vi "makeLines.vi"(7 "d (mm)":dbl, 8 "error in (no error)":errorcluster, 9 "L (mm)":dbl, 10 "N Cycles":i32, 11 "VISA Refnum in":refnum<visa-resource-name>) -> (0 "error out":errorcluster, 3 "VISA Refnum out":refnum<visa-resource-name>)   [LabVIEW 2014]
doc: "Newport Motion Controler\nThis sub VI make lines structure\n\nAndré Romero - 2022\nandretec@ifsc.usp.br"
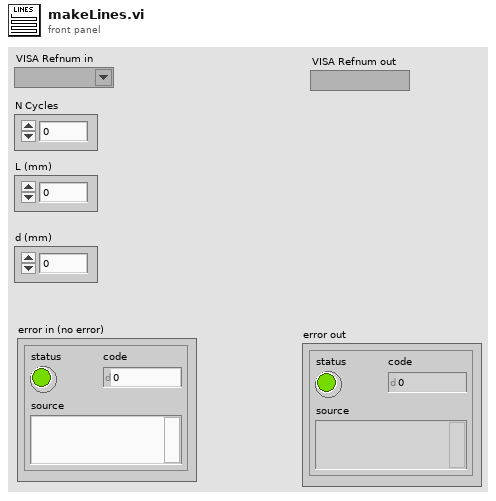
[diagram p1: front panel]
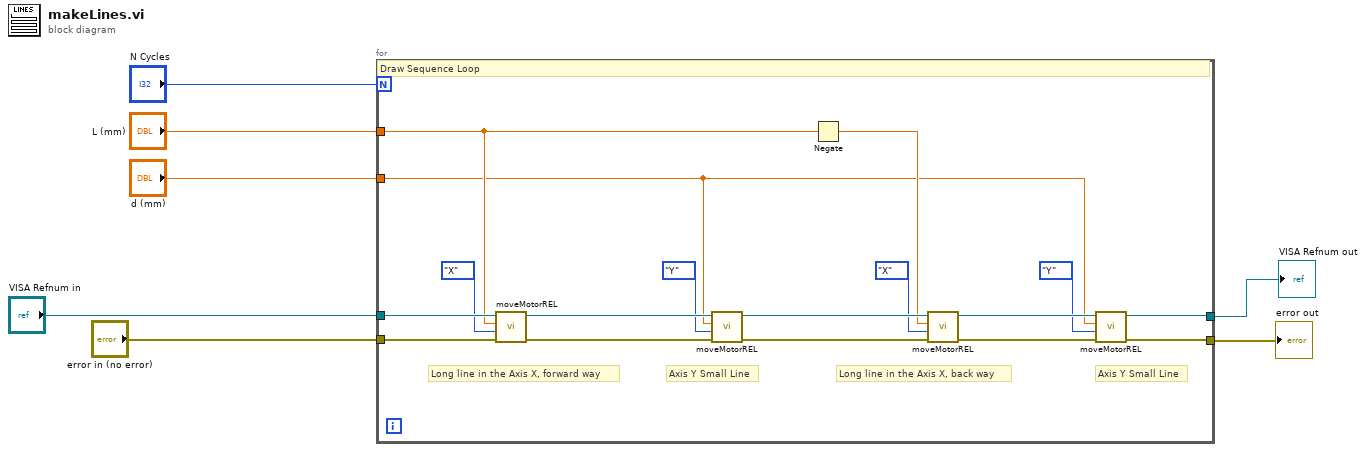
[diagram p0: block diagram]
diagram:
  n1 = for {
    N: "N Cycles" -> [_]
    tunnel: "VISA Refnum in" -> [w24]
    tunnel: "error in (no error)" -> [w23]
    tunnel: [w11] -> w1
    tunnel: [w10] -> w5
    tunnel: "L (mm)" -> [w9]
    tunnel: "d (mm)" -> [w8]
    # "Axis Y Small Line"
    # "Long line in the Axis X, back way"
    # "Axis Y Small Line"
    # "Long line in the Axis X, forward way"
    # "Draw Sequence Loop"
    n2 = call "moveMotorREL.vi"("error in (no error)"=w23, "Axis"=enum16{"X", "Y"}."X", "L (mm)"=w9, "VISA Refnum in"=w24) -> ("error out"=w20:errorcluster, "VISA Refnum out"=w21:refnum<visa-resource-name>)  [unwired: 6 in]
    n3 = call "moveMotorREL.vi"("error in (no error)"=w20, "Axis"=enum16{"X", "Y"}."Y", "L (mm)"=w8, "VISA Refnum in"=w21) -> ("error out"=w17:errorcluster, "VISA Refnum out"=w18:refnum<visa-resource-name>)  [unwired: 6 in]
    n4 = Negate(x=w9) -> (-x=w16:dbl)
    n5 = call "moveMotorREL.vi"("error in (no error)"=w17, "Axis"=enum16{"X", "Y"}."X", "L (mm)"=w16, "VISA Refnum in"=w18) -> ("error out"=w13:errorcluster, "VISA Refnum out"=w14:refnum<visa-resource-name>)  [unwired: 6 in]
    n6 = call "moveMotorREL.vi"("error in (no error)"=w13, "Axis"=enum16{"X", "Y"}."Y", "L (mm)"=w8, "VISA Refnum in"=w14) -> ("error out"=w10:errorcluster, "VISA Refnum out"=w11:refnum<visa-resource-name>)  [unwired: 6 in]
  }
  "error out" <- w5
  "VISA Refnum out" <- w1
